vi "Exp_CCD_SetExposureTime.vi"(8 "error in (no error)":errorcluster, 10 "Exposure Time (s)":dbl, 11 "LightField Automation in":refnum<class "LightField Automation.lvclass">) -> (0 "error out":errorcluster, 3 "LightField Automation out":refnum<class "LightField Automation.lvclass">)   [LabVIEW 2015, in "LightField Automation.lvclass"]
uses:
  LightField Automation.lvclass
  C:/Program Files/Princeton Instruments/LightField/PrincetonInstruments.LightFieldAddInSupportServices.dll
  Program Files/Princeton Instruments/LightField/PrincetonInstruments.LightFieldAddInSupportServices.dll
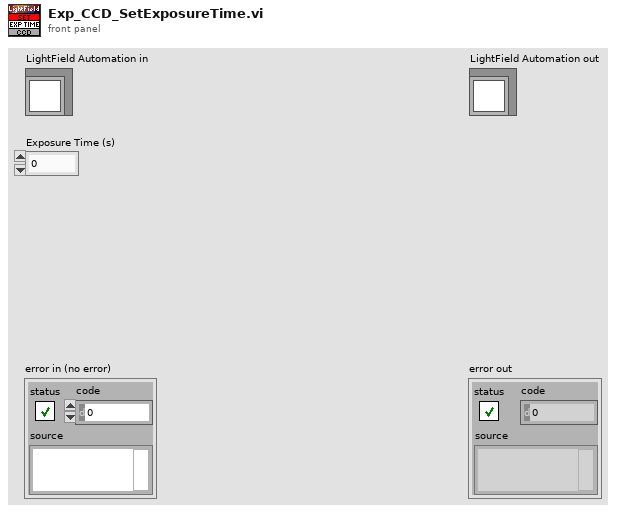
[diagram p1: front panel]
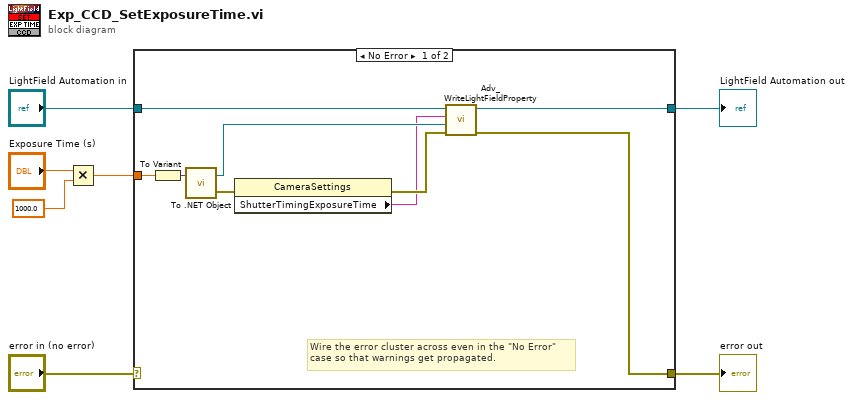
[diagram p0: block diagram]
diagram:
  n1 = Multiply(x="Exposure Time (s)", y=1000.0) -> (x*y=w1:dbl)
  n2 = case shown="No Error" "error in (no error)" {
    selector: "error in (no error)" -> [_ w18]
    tunnel: [w8 w18] -> w6
    tunnel: [w13 w17] -> w4
    tunnel: "LightField Automation in" -> [w14 w17]
    tunnel: w1 -> [w16 _]
    frame No Error {
      # "Wire the error cluster across even in the \"No Error\"\ncase so that warnings get propagated."
      n3 = To Variant(anything=w16) -> (Variant=w15:variant)
      n4 = call <vilib>:"To .NET Object.vi"("anything"=w15) -> ("error out"=w11:errorcluster, ".NET object"=w12:refnum<k24>)  [unwired: 1 in]
      n5 = property class="CameraSettings"(error in=w11) -> (error out=w10:errorcluster, "ShutterTimingExposureTime"=w9:string)  [unwired: 1 in, 1 out]
      n6 = call "Adv_WriteLightFieldProperty.vi"("error in (no error)"=w10, "value"=w12, "setting"=w9, "LightField Automation in"=w14) -> ("error out"=w8:errorcluster, "LightField Automation out"=w13:refnum<class "LightField Automation.lvclass">)  [unwired: 6 in]
    }
    frame Error {
    }
  }
  "error out" <- w6
  "LightField Automation out" <- w4
